vi "update_two_attribute_cmdlist.vi"(5 "Add to Cmd Pool":refnum<vi>, 7 "Delete from Cmd Pool":refnum<vi>, 9 "Row Index":i32) -> ()   [LabVIEW 2018]
doc: "Delete the indexed element from \"Delete from Cmd Pool\", and add the element to \"Add to Cmd Pool\"."
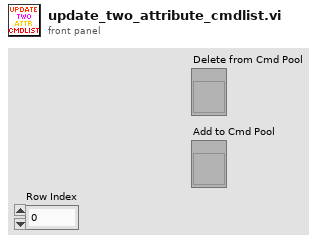
[diagram p1: front panel]
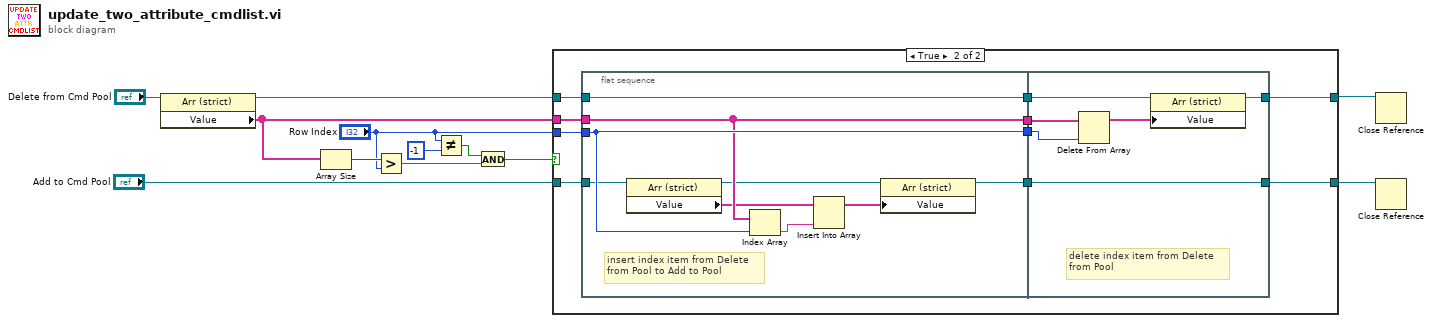
[diagram p0: block diagram]
diagram:
  n1 = property class="Arr (strict)"(reference="Delete from Cmd Pool") -> (reference out=w10:refnum<vi>, "Value"=w9:string[])  [unwired: 1 in, 1 out]
  n2 = Array Size(array=w9) -> (size(s)=w12:i32)
  n3 = Greater?(x=w12, y="Row Index") -> (0:w4:bool)
  n4 = Not Equal?(x="Row Index", y=-1) -> (x != y?=w7:bool)
  n5 = And(x=w7, y=w4) -> (x .and. y?=w3:bool)
  n6 = case shown="True" w3 {
    tunnel: w10 -> [w14 w22]
    tunnel: "Add to Cmd Pool" -> [w13 w21]
    tunnel: "Row Index" -> [_ w20]
    tunnel: [w13 w15] -> w1
    tunnel: [w14 w16] -> w2
    tunnel: w9 -> [_ w19]
    frame False {
    }
    frame True {
      n7 = flat-sequence {
        tunnel: w22 -> [w33]
        tunnel: w21 -> [w29]
        tunnel: w20 -> [w32]
        tunnel: [w33] -> w24
        tunnel: [w32] -> w23
        tunnel: w19 -> [w30]
        tunnel: [w30] -> w18
        tunnel: [w25] -> w17
        tunnel: w24 -> [w37]
        tunnel: w23 -> [w39]
        tunnel: w18 -> [w38]
        tunnel: w17 -> [w34]
        tunnel: [w35] -> w16
        tunnel: [w34] -> w15
        frame #0 {
          # "insert index item from Delete \nfrom Pool to Add to Pool"
          n8 = property class="Arr (strict)"(reference=w29) -> (reference out=w27:refnum<vi>, "Value"=w28:string[])  [unwired: 1 in, 1 out]
          n9 = Index Array(array=w30, index=w32) -> (element=w31:string)
          n10 = Insert Into Array(array=w28, new element=w31) -> (w26:string[])  [unwired: 1 in]
          n11 = property class="Arr (strict)"(reference=w27, "Value"=w26) -> (reference out=w25:refnum<vi>)  [unwired: 1 in, 1 out]
        }
        frame #1 {
          # "delete index item from Delete \nfrom Pool"
          n12 = Delete From Array(array=w38, index=w39) -> (array with subset deleted=w36:string[])  [unwired: 1 in, 1 out]
          n13 = property class="Arr (strict)"(reference=w37, "Value"=w36) -> (reference out=w35:refnum<vi>)  [unwired: 1 in, 1 out]
        }
      }
    }
  }
  n14 = Close Reference(reference=w2) -> ()  [unwired: 1 in, 1 out]
  n15 = Close Reference(reference=w1) -> ()  [unwired: 1 in, 1 out]
